vi "Host_SimulateData.vi"() -> ()   [LabVIEW 2017]
doc: "Dialogue window to allow user to manually upload/override/simulate data normally aquired by cRIO.\nCalled by pressing \"Simulate Data\" button on front panel of Host__Main.vi"
uses:
  Master/DAQ/Master_DataControl.ctl
  Master/DAQ/TypeDef_cRIOData.ctl
  Master/IMU/TypeDef_IMUData.ctl
  Master/CAN/TypeDef_BMSData.ctl
  Master/CAN/TypeDef_BMS_Status.ctl
  Master/CAN/MotorController/fixedMotorData.ctl
  Master/CAN/MotorController/MotorStatus.ctl
panel:
  in  "DataOverride":T1={"cRIO Data"={"Time (ms)"=0.0, "24V Battery (V)"=26.0, "LowV Current (A)"=2.5, "Fiducial Sensor (V)"=0.0, "PV Pressure (psig)"=15.0, "Flow Sensor (V)"=0.0, "Temp Fairing (F)"=0.0, "Temp Reservoir (F)"=0.0, "HallEffect Right (in)"=1.85, "HallEffect Left (in)"=1.85, "PT Tank (psig)"=2000.0, "PT Clamp Right (psig)"=12.5, "PT Clamp Left (psig)"=12.5, "PT Brake (psig)"=30.0, "PT Cooling (psig)"=15.0, "Displacement (ft)"=0.0, "Velocity (ft/s)"=0.0}, "IMU Data"={"x acceleration (g)"=0.0, "Pressure (psia)"=15.0, "Temperature (F)"=80.0}, "BMS Data"={"Max Cell Voltage (V)"=4.0, "Max Cell ID"=0.0, "Min Cell Voltage (V)"=3.9, "Min Cell ID"=0.0, "State of Charge (%)"=50.0, "Average Voltage (V)"=0.0, "Voltage Delta (V)"=0.0, "Pack Current (A)"=0.0, "Pack Voltage (V)"=0.0, "Max Resistance (Ohm)"=0.0, "Min Resistance (Ohm)"=0.0, "Average Resistance (Ohm)"=0.0, "Delta Resistance (Ohm)"=0.0, "Highest Temperature(F)"=80.0, "BmsStatus"={"isFault"=FALSE, "isolationMonitoring"=FALSE}}, "Motor Data"={"Velo (RPM)"=0.0, "MotorTemp(F)"=0.0, "CtrlTemp(F)"=0.0, "DcLinkVolt(V)"=0.0, "ErrorCode"=0.0, "motorStatus"={"isReady"=FALSE, "isOn"=FALSE, "isOperEn"=FALSE, "isFault"=FALSE, "isVoltEn"=FALSE, "targetReached"=FALSE, "isWarning"=FALSE}, "isAlive"=FALSE, "motorControllerState"=1}} {"Motor Data"."motorControllerState" items=["unknown"=1, "boot-up"=0, "stopped"=4, "operational"=5, "pre-operational"=127, "connection lost"=128]}
  in  "Process Stop Button":bool
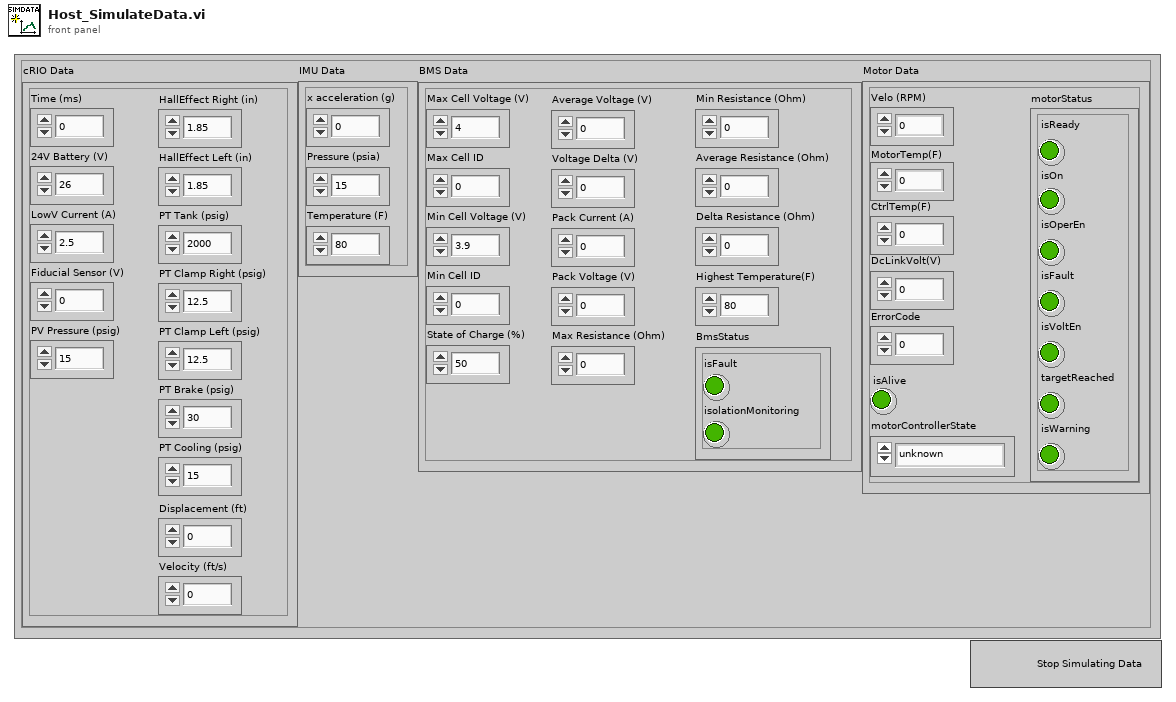
[diagram p1: front panel]
types:
  T1 = typedef "Master_DataControl.ctl" = cluster{"cRIO Data":T2, "IMU Data":T3, "BMS Data":T4, "Motor Data":T6}
  T2 = typedef "TypeDef_cRIOData.ctl" = cluster{"Time (ms)":dbl, "24V Battery (V)":dbl, "LowV Current (A)":dbl, "Fiducial Sensor (V)":dbl, "PV Pressure (psig)":dbl, "Flow Sensor (V)":dbl, "Temp Fairing (F)":dbl, "Temp Reservoir (F)":dbl, "HallEffect Right (in)":dbl, "HallEffect Left (in)":dbl, "PT Tank (psig)":dbl, "PT Clamp Right (psig)":dbl, "PT Clamp Left (psig)":dbl, "PT Brake (psig)":dbl, "PT Cooling (psig)":dbl, "Displacement (ft)":dbl, "Velocity (ft/s)":dbl}
  T3 = typedef "TypeDef_IMUData.ctl" = cluster{"x acceleration (g)":dbl, "Pressure (psia)":dbl, "Temperature (F)":dbl}
  T4 = typedef "TypeDef_BMSData.ctl" = cluster{"Max Cell Voltage (V)":dbl, "Max Cell ID":dbl, "Min Cell Voltage (V)":dbl, "Min Cell ID":dbl, "State of Charge (%)":dbl, "Average Voltage (V)":dbl, "Voltage Delta (V)":dbl, "Pack Current (A)":dbl, "Pack Voltage (V)":dbl, "Max Resistance (Ohm)":dbl, "Min Resistance (Ohm)":dbl, "Average Resistance (Ohm)":dbl, "Delta Resistance (Ohm)":dbl, "Highest Temperature(F)":dbl, "BmsStatus":T5}
  T5 = typedef "TypeDef_BMS_Status.ctl" = cluster{"isFault":bool, "isolationMonitoring":bool}
  T6 = typedef "fixedMotorData.ctl" = cluster{"Velo (RPM)":dbl, "MotorTemp(F)":dbl, "CtrlTemp(F)":dbl, "DcLinkVolt(V)":dbl, "ErrorCode":dbl, "motorStatus":T7, "isAlive":bool, "motorControllerState":u16}
  T7 = typedef "MotorStatus.ctl" = cluster{"isReady":bool, "isOn":bool, "isOperEn":bool, "isFault":bool, "isVoltEn":bool, "targetReached":bool, "isWarning":bool}
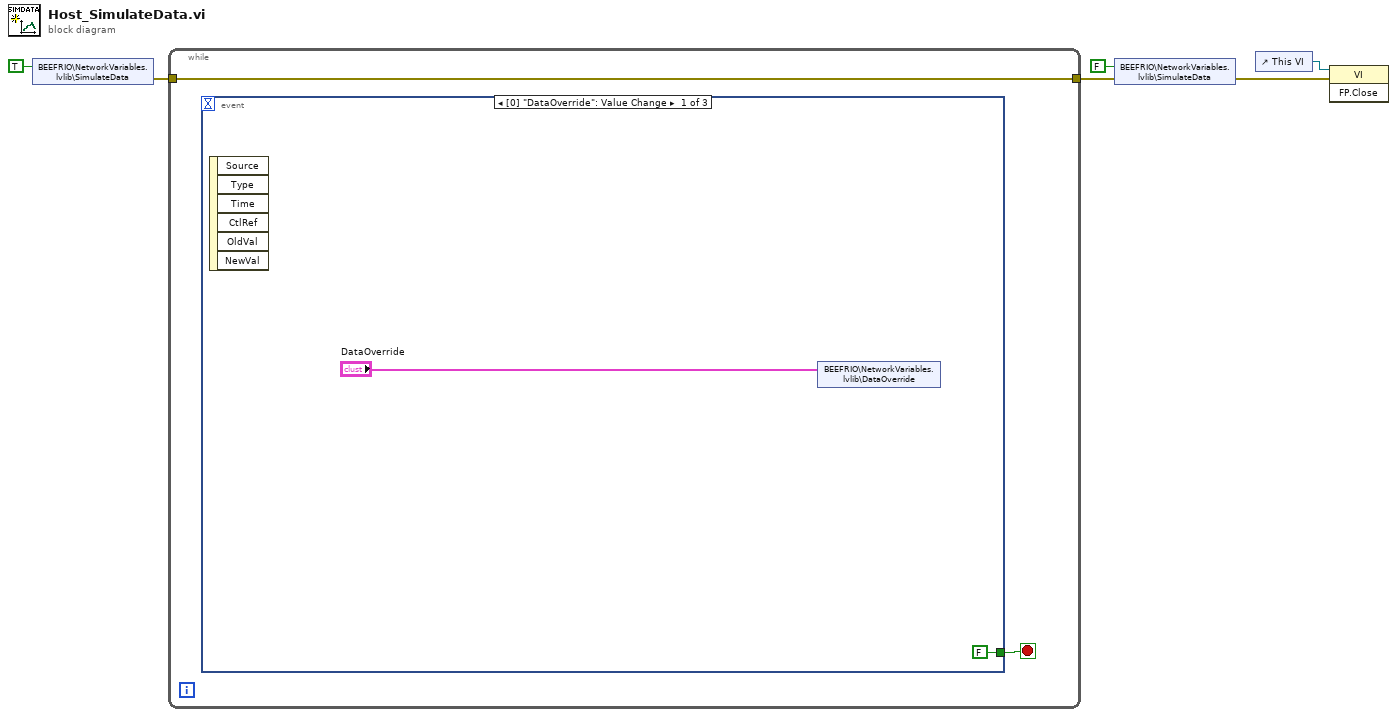
[diagram p0: block diagram]
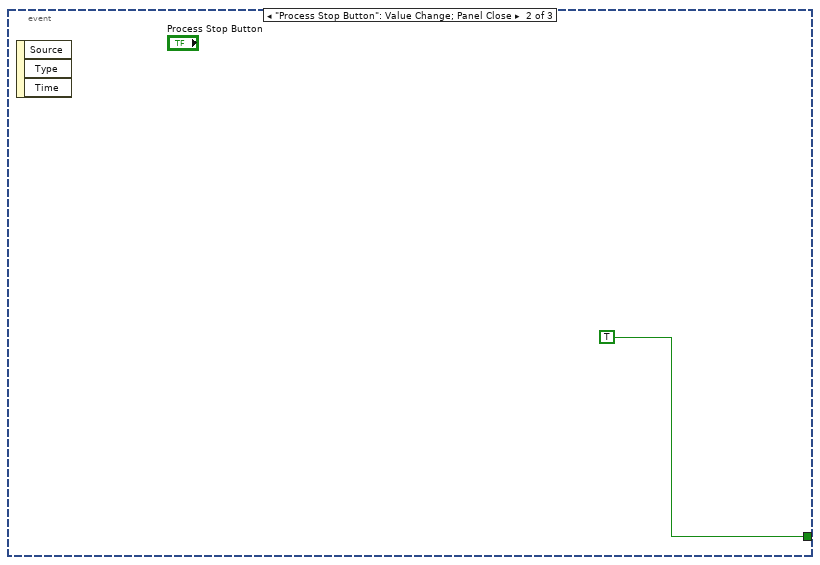
[diagram p2: hidden frame]
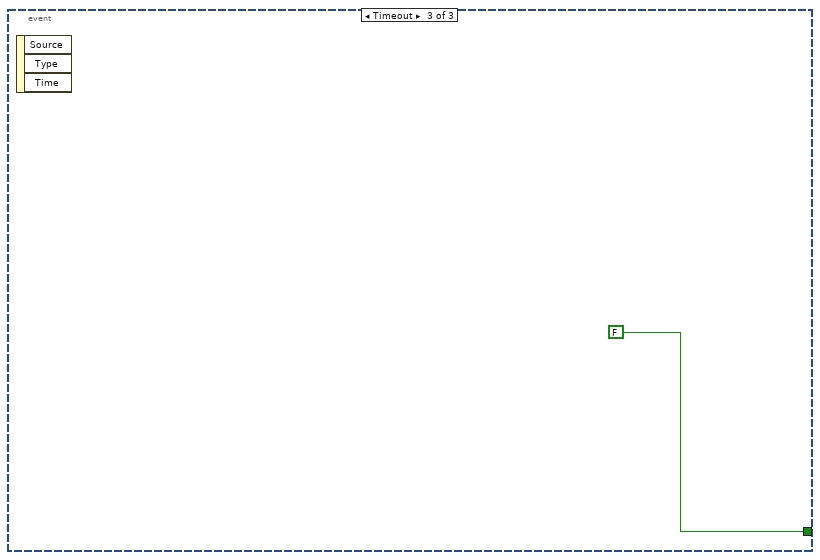
[diagram p3: hidden frame]
diagram:
  n1 = shared-variable "BEEFRIO\\NetworkVariables.lvlib\\SimulateData"(TRUE ("SimulateData")) -> (error out=w5:errorcluster)  [unwired: 1 in]
  n2 = while {
    tunnel: w5 -> [w7]
    tunnel: [w7] -> w3
    stop <- w8 stop-if-true
    n3 = event shown="[0] \"DataOverride\": Value Change" {
      selector: _ -> [_ _ _]
      dyn-events: _ -> [_ _ _]
      timeout: _ -> [_ _ _]
      tunnel: [FALSE TRUE FALSE] -> w8
      event Value Change {
        n4 = event-data() -> ()  [unwired: 1 in, 6 out]
        n5 = shared-variable "BEEFRIO\\NetworkVariables.lvlib\\DataOverride"("DataOverride") -> ()  [unwired: 1 in, 1 out]
      }
      event "Process Stop Button": Value Change; Panel Close {
        n6 = event-data() -> ()  [unwired: 1 in, 3 out]
      }
      event Timeout {
        n7 = event-data() -> ()  [unwired: 1 in, 3 out]
      }
    }
  }
  n8 = shared-variable "BEEFRIO\\NetworkVariables.lvlib\\SimulateData"(FALSE ("SimulateData"), error in=w3) -> (error out=w2:errorcluster)
  n9 = control-ref of="This VI"() -> (w1:refnum<vi>)
  n10 = invoke class="VI" method="FP.Close"(reference=w1, error in=w2) -> ()  [unwired: 1 in, 3 out]
